vi "test - Cluster2.vi"(8 "error in (no error)":errorcluster, 11 "TestCase in":refnum<class "testcase-Supported-Datatype.lvclass">) -> (0 "error out":errorcluster, 3 "TestCase out":refnum<class "testcase-Supported-Datatype.lvclass">)   [LabVIEW 2017, in "testcase-Supported-Datatype.lvclass"]
uses:
  testcase-Supported-Datatype.lvclass
  f1af1619-b1ee-4d97-8553-569f79cc2304.vi
  101d9ff8-76c4-4606-8f2f-ee3dde8ae347.vi
  2ea916dd-69fc-4974-898a-c6913463711b.vi
  addons/API-String-Arugments-Support/_Support/Convert API String Arguments to Data(variant).vi
  addons/API-String-Arugments-Support/_Support/Data To API String Arguments.vi
  <vilib>/addons/_JKI Toolkits/VI Tester/TestCase.llb/TestCase.lvclass
  C:/Program Files (x86)/National Instruments/LabVIEW 2017/vi.lib/addons/_JKI Toolkits/VI Tester/TestCase.llb/TestCase.lvclass
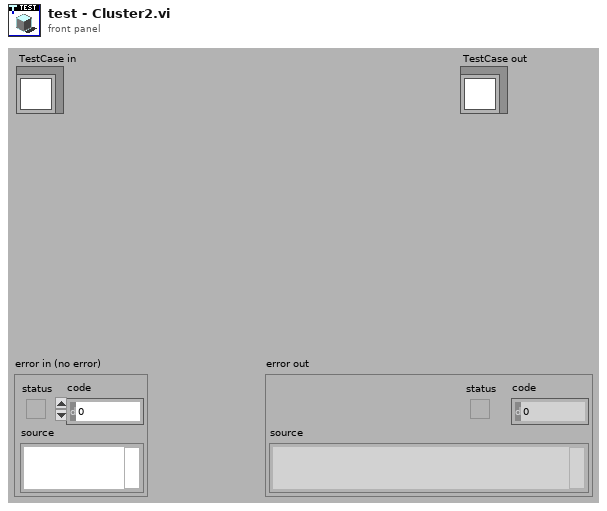
[diagram p1: front panel]
types:
  T1 = cluster{"Name":string, "Child":cluster{"Name":string}, "Bool":bool}
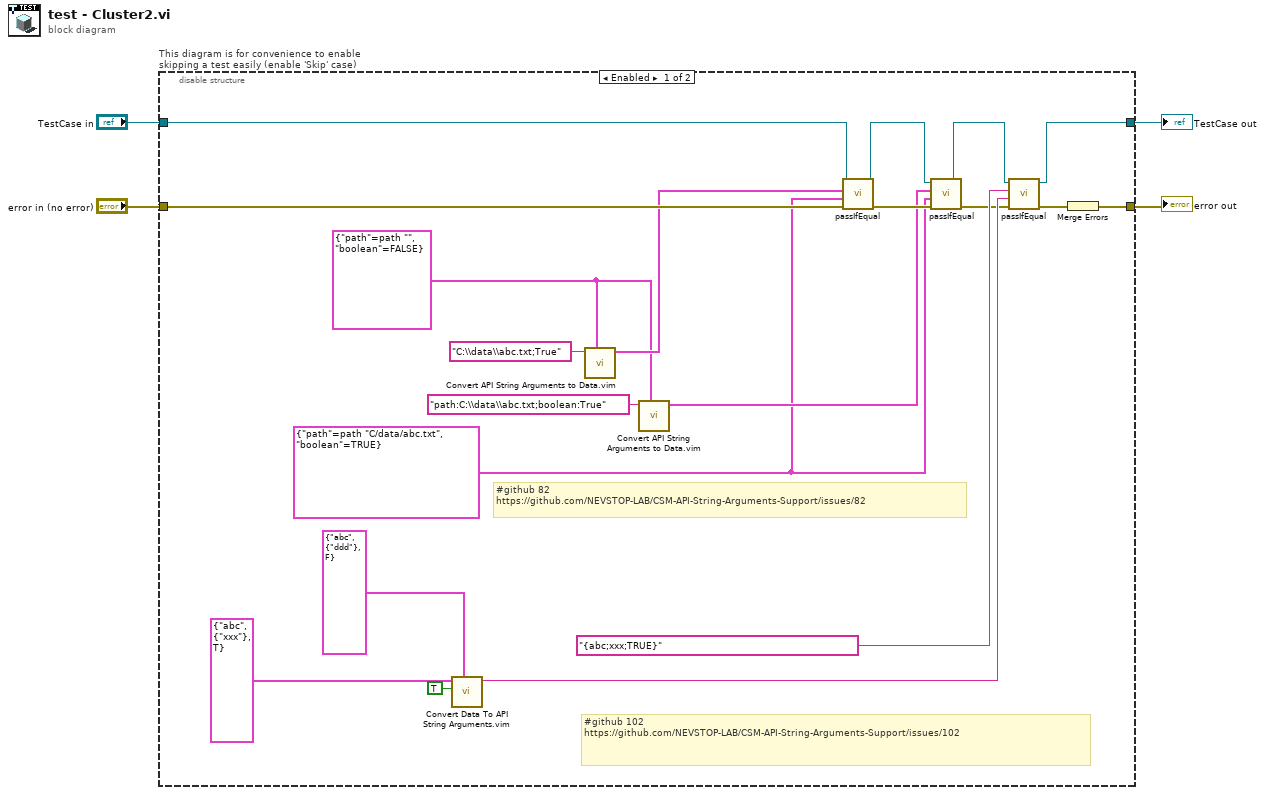
[diagram p0: block diagram]
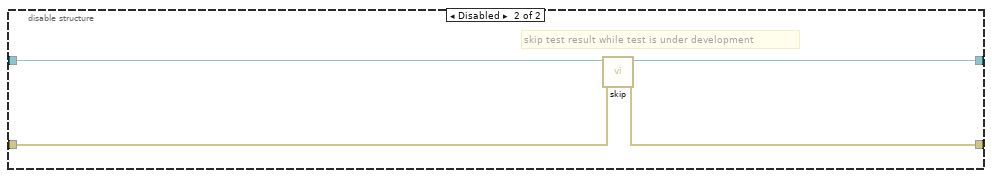
[diagram p2: hidden frame]
diagram:
  n1 = disable-structure "This diagram is for convenience to enable skipping a test easily (enable 'Skip' case)" shown="Enabled" {
    disable-tunnel: "TestCase in" -> [w24 w28]
    disable-tunnel: [w9 w26] -> w1
    disable-tunnel: [w22 w27] -> w3
    disable-tunnel: "error in (no error)" -> [w23 w25]
    frame Enabled {
      w16 = cluster{"path":path, "boolean":bool} {"path"=path "", "boolean"=FALSE}
      w14 = cluster{"path":path, "boolean":bool} {"path"=path "C:/data/abc.txt", "boolean"=TRUE}
      # "#github 102\nhttps://github.com/NEVSTOP-LAB/CSM-API-String-Arguments-Support/issues/102"
      # "#github 82\nhttps://github.com/NEVSTOP-LAB/CSM-API-String-Arguments-Support/issues/82"
      n2 = call "Convert Data To API String Arguments.vim"("Reference Cluster Data"=T1 {"Name"="abc", "Child"={"Name"="ddd"}, "Bool"=FALSE} ("Reference cluster data"), "No Tag Mode? (F)"=TRUE ("No Tag Mode(F)"), "Data"=T1 {"Name"="abc", "Child"={"Name"="xxx"}, "Bool"=TRUE} ("Data 8")) -> ("API String"=w8:string)  [unwired: 5 in, 1 out]
      n3 = call "Convert API String Arguments to Data.vim"("Reference Type"=w16, "API String"="C:\\data\\abc.txt;True" ("String")) -> ("Data"=w21:cluster{"path":path, "boolean":bool})  [unwired: 6 in, 1 out]
      n4 = call "Convert API String Arguments to Data.vim"("Reference Type"=w16, "API String"="path:C:\\data\\abc.txt;boolean:True" ("String")) -> ("Data"=w15:cluster{"path":path, "boolean":bool})  [unwired: 6 in, 1 out]
      n5 = call-dynamic "passIfEqual.vi"("error in (no error)"=w23, "y"=w14, "x"=w21, "TestCase in"=w24) -> ("error out"=w18:errorcluster, "TestCase out"=w19:refnum<class "testcase-Supported-Datatype.lvclass">)  [unwired: 6 in]
      n6 = call-dynamic "passIfEqual.vi"("error in (no error)"=w18, "y"=w14, "x"=w15, "TestCase in"=w19) -> ("error out"=w5:errorcluster, "TestCase out"=w10:refnum<class "testcase-Supported-Datatype.lvclass">)  [unwired: 6 in]
      n7 = call-dynamic "passIfEqual.vi"("error in (no error)"=w5, "y"=w8, "x"="{abc;xxx;TRUE}" ("String"), "TestCase in"=w10) -> ("error out"=w6:errorcluster, "TestCase out"=w9:refnum<class "testcase-Supported-Datatype.lvclass">)  [unwired: 6 in]
      n8 = Merge Errors(w6) -> (w22:errorcluster)
    }
    frame Disabled {
      # "skip test result while test is under development"
      n9 = call <vilib>:"skip.vi"("error in (no error)"=w25, "TestCase in"=w28) -> ("error out"=w27:errorcluster, "TestCase out"=w26:refnum<class "testcase-Supported-Datatype.lvclass">)  [unwired: 8 in]
    }
  }
  "error out" <- w3
  "TestCase out" <- w1
